vi "SCADA.vi"() -> ()   [LabVIEW 2014]
uses:
  <vilib>/platform/TimedLoop/XDataNode/XDataNode.xnode
  <vilib>/Platform/TimedLoop/XDataNode/nitl_modes.ctl
  <vilib>/Platform/TimedLoop/XDataNode/XDNodeRunTimeDep.lvlib
  <vilib>/Platform/TimedLoop/XDataNode/wakeup.ctl
  <vilib>/Platform/TimedLoop/XDataNode/timing_clust.ctl
panel:
  out "Hand_Error":bool
  out "Tasks":string
  out "State":string
  in  "HAND/AUTO":bool=TRUE
  in  "EMERGENCY ON/OFF":bool
  out "Fault":bool
  in  "ACK FAULT":bool
  in  "PUMPS OFF":bool
  in  "PUMPS ON":bool
  in  "SYSTEM OFF":bool
  in  "SYSTEM ON":bool
  out "error IO":errorcluster
  in  "error in (no error)":errorcluster
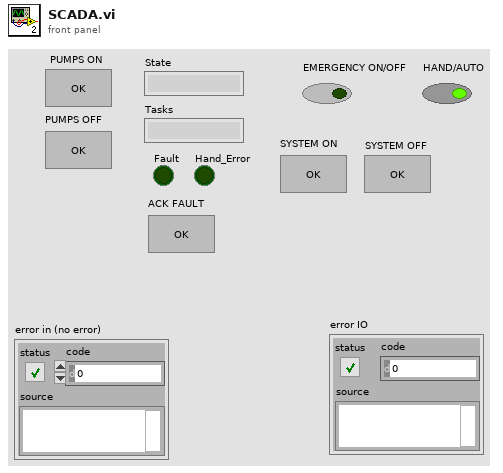
[diagram p1: front panel]
types:
  T1 = typedef "XDNodeRunTimeDep.lvlib/timing_clust.ctl" = cluster{"Expected End [f-1]":u64, "Actual End [f-1]":u64, "Finished Late? [f-1]":bool, "Expected End [i-1]":u64, "Actual End [i-1]":u64, "Finished Late? [i-1]":bool, "Expected Start [i]":u64, "Actual Start [i]":u64, "Expected Start [f]":u64, "Actual Start [f]":u64, "Source Name":string, "Structure Name":string, "Period":i64, "Deadline":i64, "Offset":i64, "Start":i64, "Priority":i32, "Timeout":i32, "Mode":T2, "Wakeup Reason":T3, "Error":errorcluster, "Source Type":string, "Secondary Source Type":string, "Global End Time":u64, "Global Start Time":u64, "Frame Duration":u64, "Iteration Duration":u64, "Assigned CPU":i32, "I/O Scan Engine Mode":u32}
  T2 = typedef "XDNodeRunTimeDep.lvlib/nitl_modes.ctl" = enum32{"No Change", "Process missed periods, maintain original phase", "Discard missed periods, maintain original phase", "Process missed periods, ignore original phase", "Discard missed periods, ignore original phase"}
  T3 = typedef "XDNodeRunTimeDep.lvlib/wakeup.ctl" = enum32{"Normal", "Aborted", "Asynchronous wakeup", "Timing source error", "Timed loop error", "Timeout"}
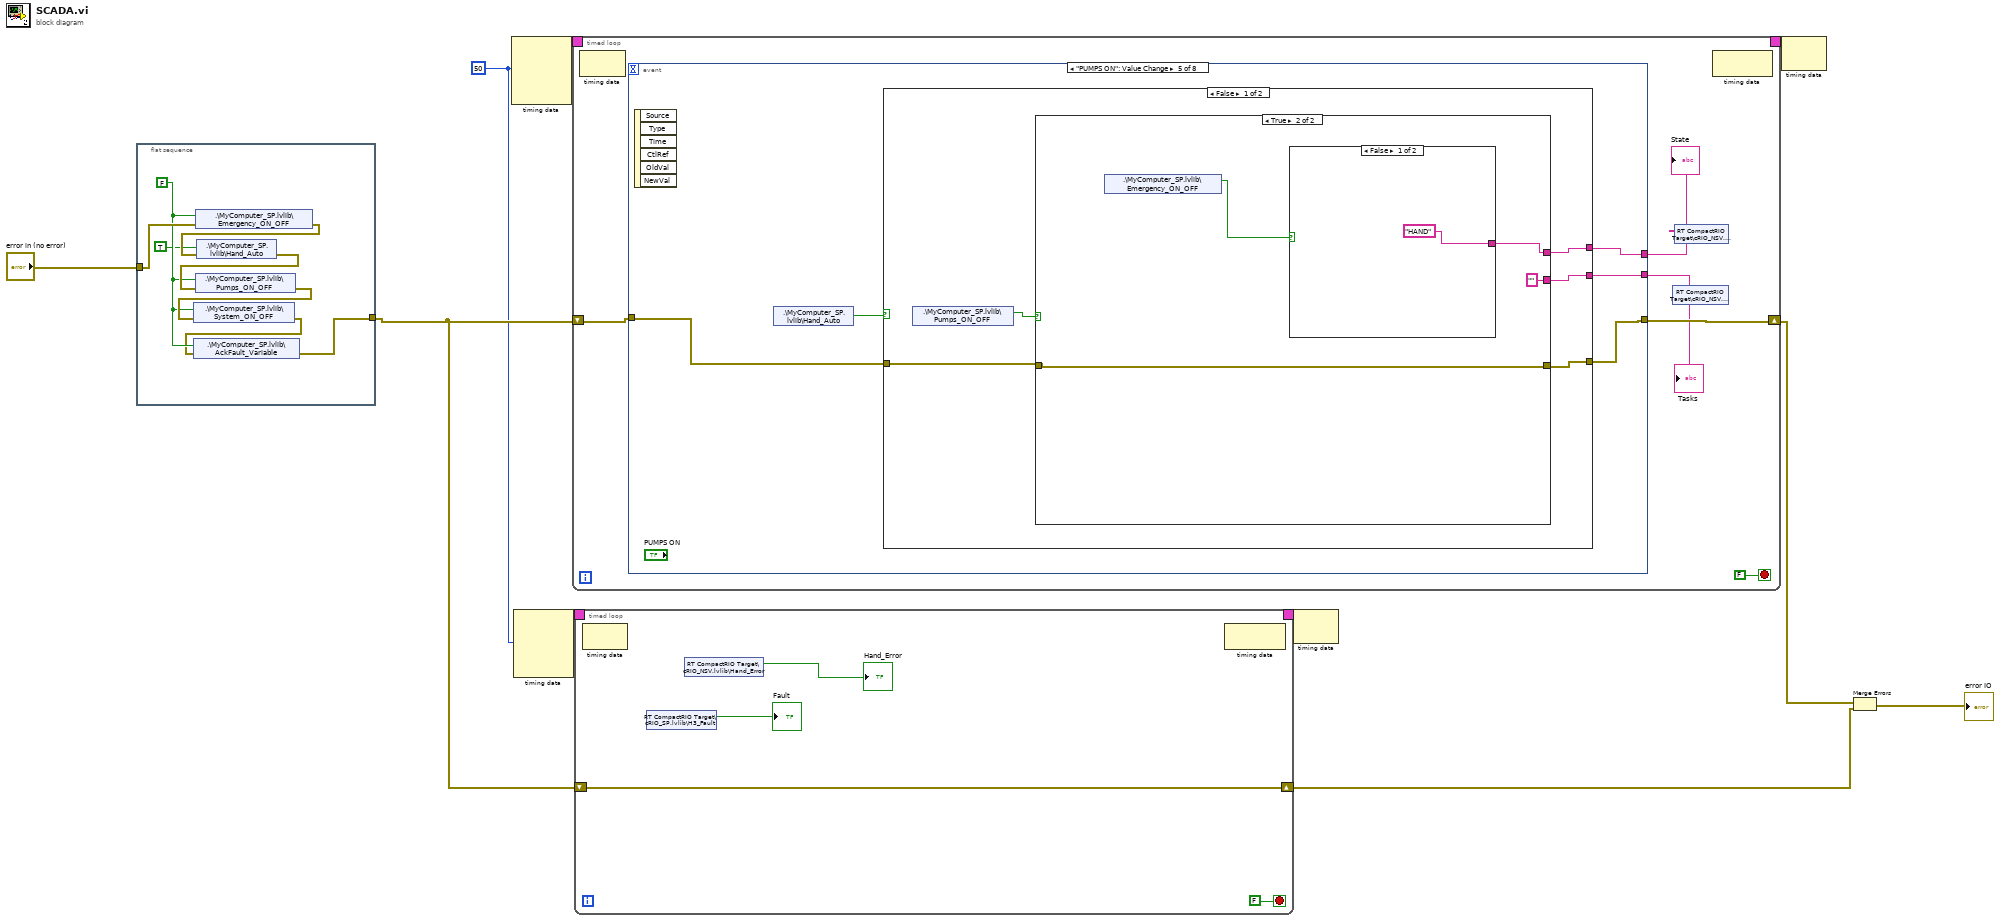
[diagram p0: block diagram]
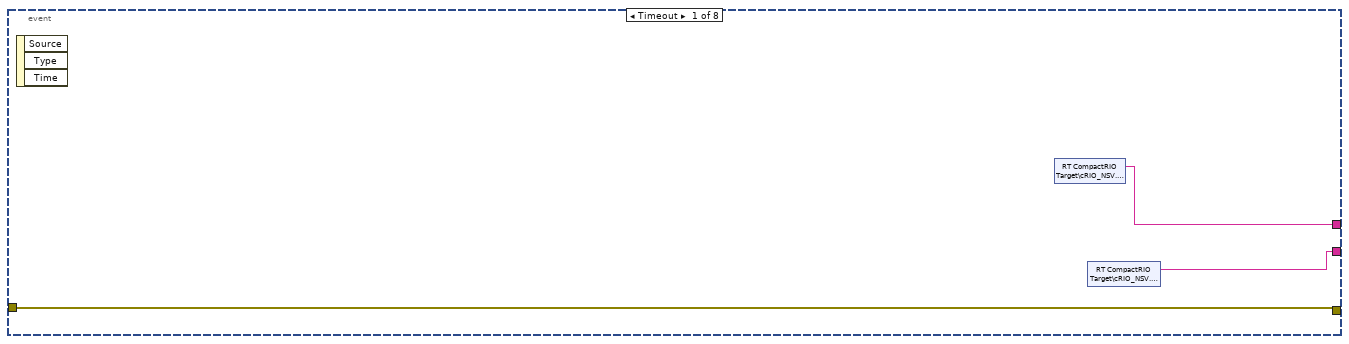
[diagram p2: hidden frame]
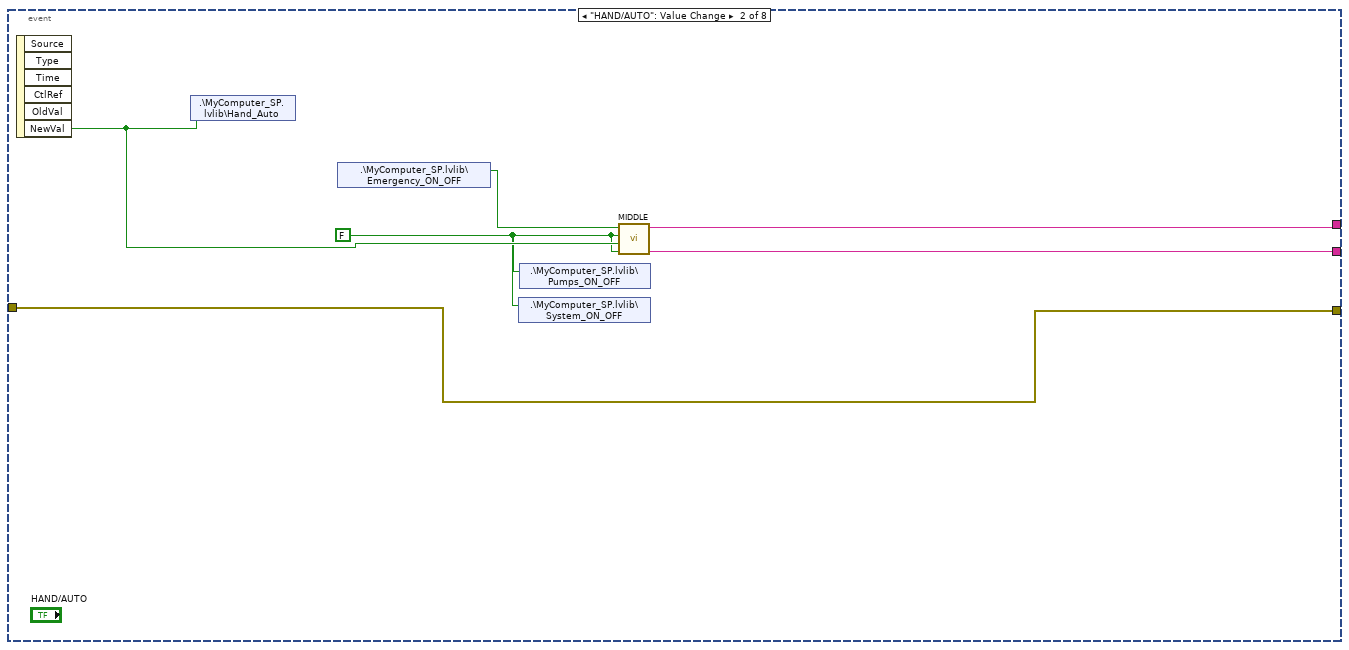
[diagram p3: hidden frame]
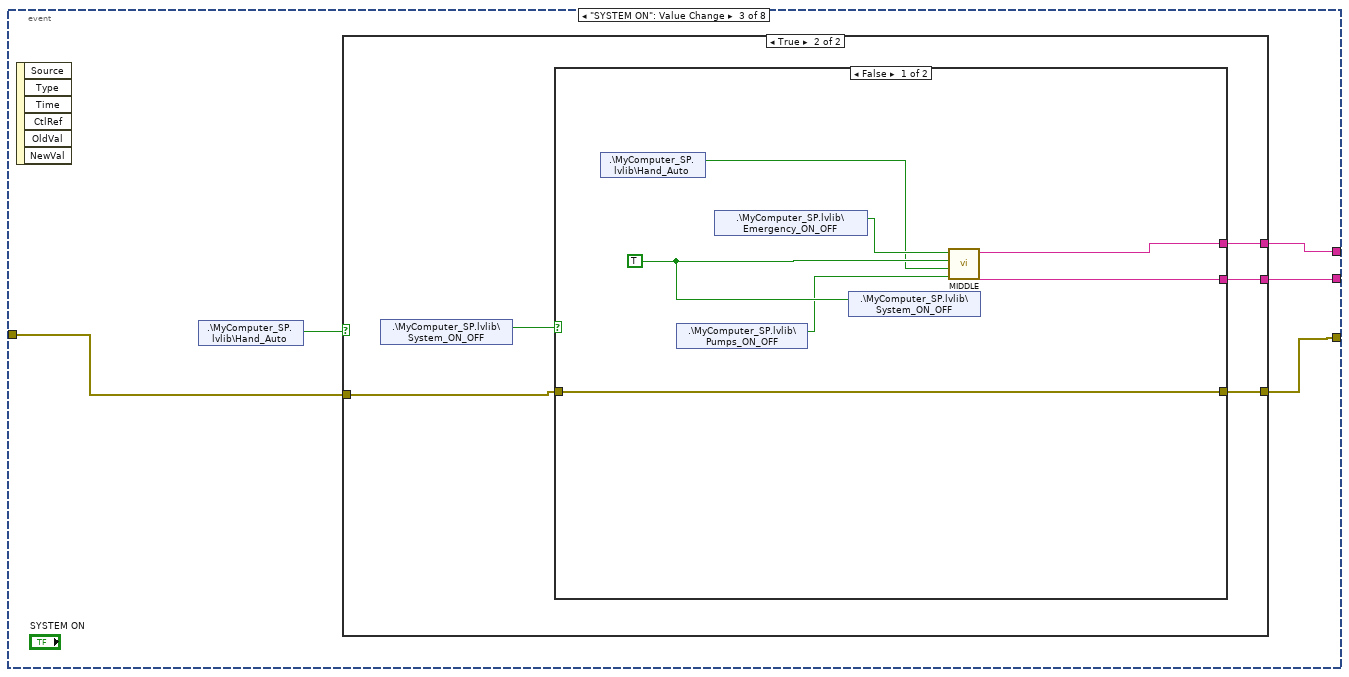
[diagram p4: hidden frame]
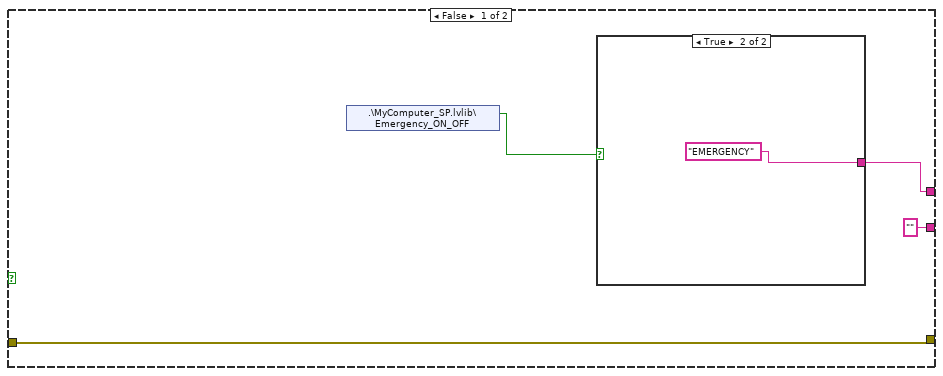
[diagram p5: hidden frame]
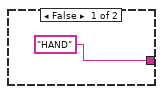
[diagram p6: hidden frame]
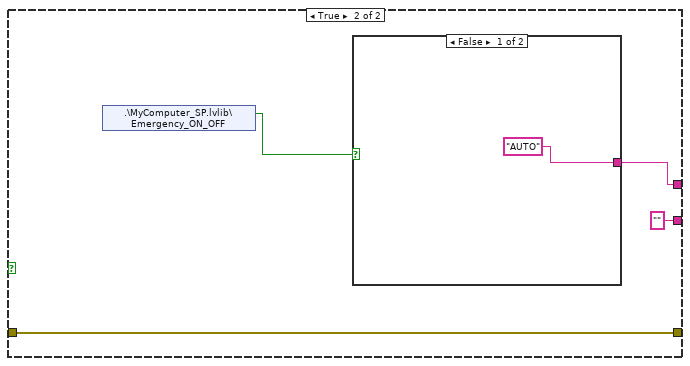
[diagram p7: hidden frame]
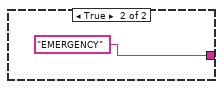
[diagram p8: hidden frame]
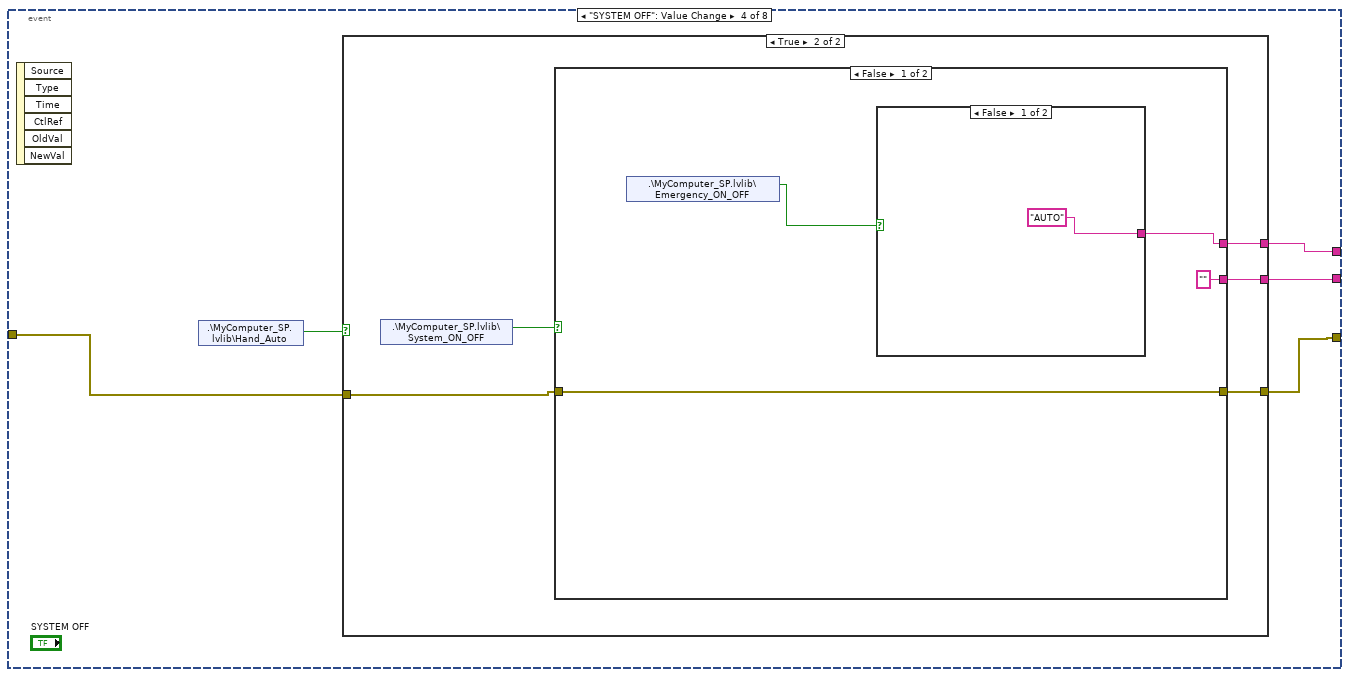
[diagram p9: hidden frame]
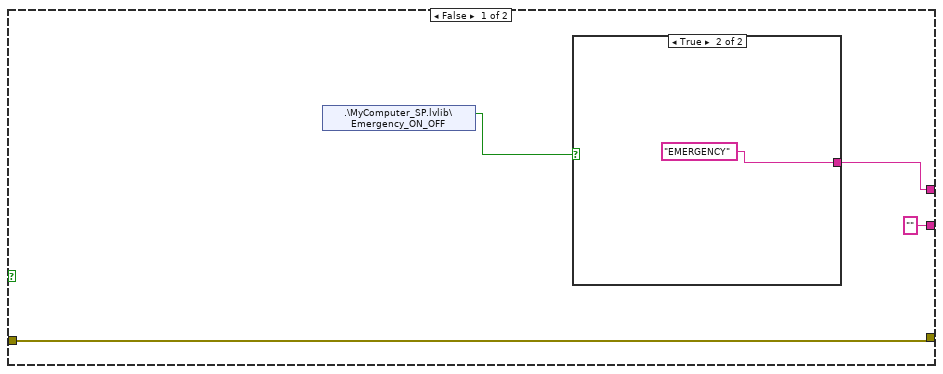
[diagram p10: hidden frame]
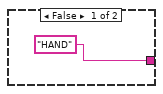
[diagram p11: hidden frame]
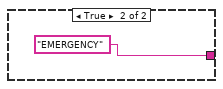
[diagram p12: hidden frame]
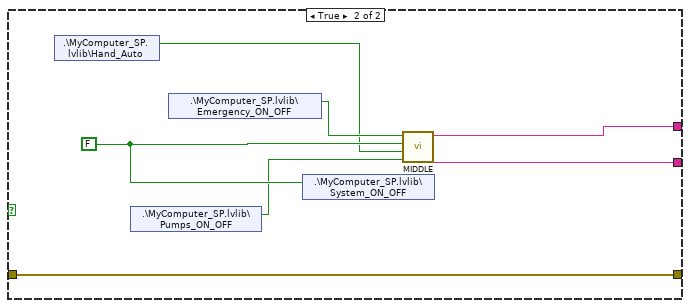
[diagram p13: hidden frame]
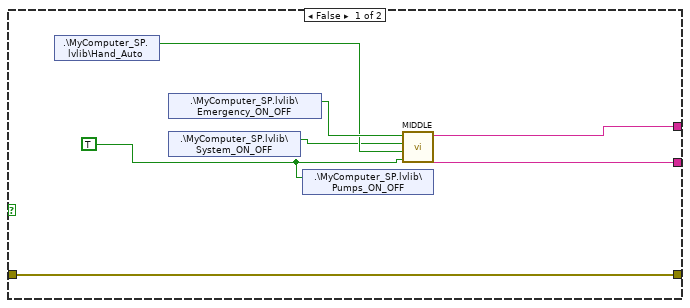
[diagram p14: hidden frame]
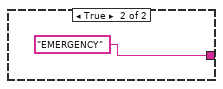
[diagram p15: hidden frame]
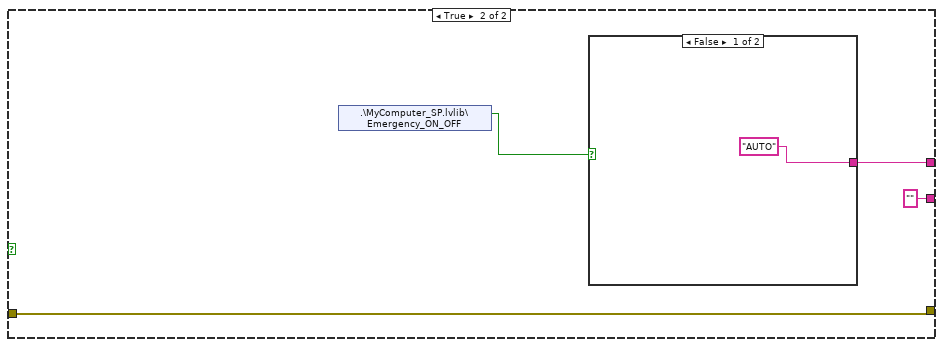
[diagram p16: hidden frame]
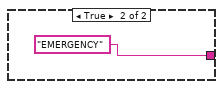
[diagram p17: hidden frame]
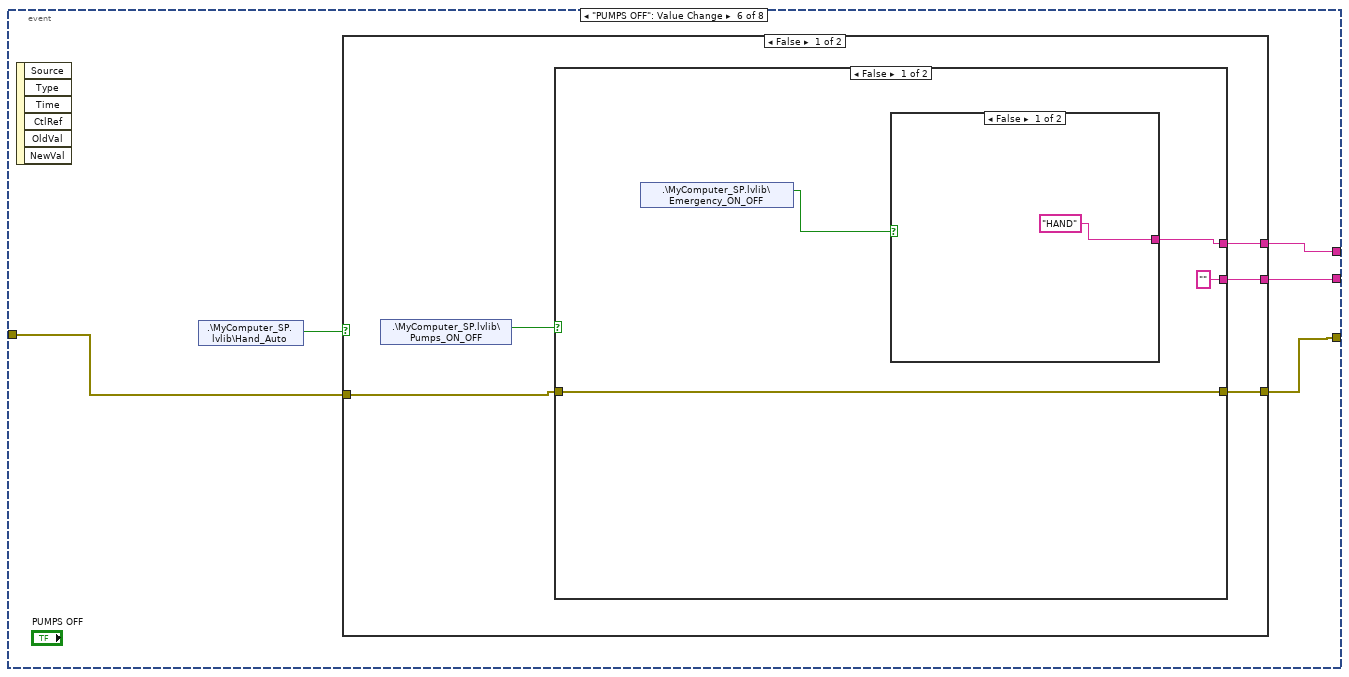
[diagram p18: hidden frame]
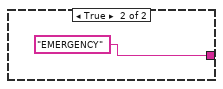
[diagram p19: hidden frame]
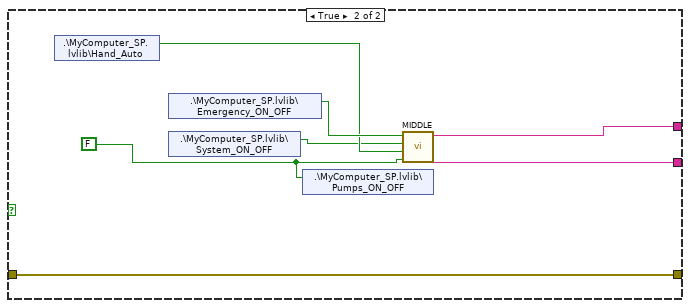
[diagram p20: hidden frame]
diagram:
  w1 = i64 50 ("Period")
  n1 = flat-sequence {
    tunnel: "error in (no error)" -> [w18]
    tunnel: [w12] -> w6
    frame #0 {
      w14 = FALSE
      n2 = shared-variable ".\\MyComputer_SP.lvlib\\Emergency_ON_OFF"(w14, error in=w18) -> (error out=w17:errorcluster)
      n3 = shared-variable ".\\MyComputer_SP.lvlib\\Hand_Auto"(TRUE, error in=w17) -> (error out=w16:errorcluster)
      n4 = shared-variable ".\\MyComputer_SP.lvlib\\Pumps_ON_OFF"(w14, error in=w16) -> (error out=w15:errorcluster)
      n5 = shared-variable ".\\MyComputer_SP.lvlib\\System_ON_OFF"(w14, error in=w15) -> (error out=w13:errorcluster)
      n6 = shared-variable ".\\MyComputer_SP.lvlib\\AckFault_Variable"(w14, error in=w13) -> (error out=w12:errorcluster)
    }
  }
  n7 = node-c288(w1) -> (w5:T1)  [unwired: 3 in]
  n8 = node-c288(w1) -> (w3:T1)  [unwired: 3 in]
  n9 = timed-loop {
    shift-right: [w21] -> w9
    shift-left: w6 -> [w22]
    timing: w5 -> [_]
    timing-out: [_] -> w4
    stop <- FALSE stop-if-true
    n10 = node-c288() -> ()  [unwired: 1 in, 1 out]
    n11 = event shown="[4] \"PUMPS ON\": Value Change" {
      selector: _ -> [_ _ _ _ _ _ _ _]
      dyn-events: _ -> [_ _ _ _ _ _ _ _]
      timeout: _ -> [_ _ _ _ _ _ _ _]
      tunnel: w22 -> [w26 w29 w36 w65 w94 w123 w152 w169]
      tunnel: [w28 w31 w37 w66 w95 w124 w154 w167] -> w20
      tunnel: [w27 w30 w38 w67 w96 w125 w153 w166] -> w19
      tunnel: [w26 w29 w35 w64 w93 w122 w151 w168] -> w21
      event Timeout {
        n12 = event-data() -> ()  [unwired: 1 in, 3 out]
        n13 = shared-variable "RT CompactRIO Target\\cRIO_NSV.lvlib\\State"() -> (w28:string)  [unwired: 1 in, 1 out]
        n14 = shared-variable "RT CompactRIO Target\\cRIO_NSV.lvlib\\Tasks"() -> (w27:string)  [unwired: 1 in, 1 out]
      }
      event "HAND/AUTO": Value Change {
        w32 = FALSE
        n15 = event-data() -> ("NewVal"=w33:bool)  [unwired: 1 in, 5 out]
        n16 = shared-variable ".\\MyComputer_SP.lvlib\\Hand_Auto"(w33) -> ()  [unwired: 1 in, 1 out]
        n17 = shared-variable ".\\MyComputer_SP.lvlib\\Emergency_ON_OFF"() -> (w34:bool)  [unwired: 1 in, 1 out]
        n18 = shared-variable ".\\MyComputer_SP.lvlib\\System_ON_OFF"(w32) -> ()  [unwired: 1 in, 1 out]
        n19 = shared-variable ".\\MyComputer_SP.lvlib\\Pumps_ON_OFF"(w32) -> ()  [unwired: 1 in, 1 out]
        n20 = call "MIDDLE.vi"("PUMPS ON/OFF"=w32, "HAND/AUTO"=w33, "SYSTEM ON/OFF"=w32, "EMERGENCY ON/OFF"=w34) -> ("Tasks"=w30:string, "State"=w31:string)  [unwired: 6 in]
      }
      event "SYSTEM ON": Value Change {
        n21 = event-data() -> ()  [unwired: 1 in, 6 out]
        n22 = shared-variable ".\\MyComputer_SP.lvlib\\Hand_Auto"() -> (w39:bool)  [unwired: 1 in, 1 out]
        n23 = case shown="True" w39 {
          tunnel: ["" ("String") w49] -> w38
          tunnel: [w40 w48] -> w37
          tunnel: w36 -> [w43 w47]
          tunnel: [w43 w46] -> w35
          frame False {
            n24 = shared-variable ".\\MyComputer_SP.lvlib\\Emergency_ON_OFF"() -> (w41:bool)  [unwired: 1 in, 1 out]
            n25 = case shown="True" w41 {
              tunnel: ["HAND" ("String") "EMERGENCY" ("String")] -> w40
              frame False {
              }
              frame True {
              }
            }
          }
          frame True {
            n26 = shared-variable ".\\MyComputer_SP.lvlib\\System_ON_OFF"() -> (w50:bool)  [unwired: 1 in, 1 out]
            n27 = case shown="False" w50 {
              tunnel: [w52 "" ("Tasks")] -> w49
              tunnel: [w53 w58] -> w48
              tunnel: w47 -> [w51 w61]
              tunnel: [w51 w61] -> w46
              frame False {
                w56 = TRUE ("SYSTEM ON/OFF")
                n28 = shared-variable ".\\MyComputer_SP.lvlib\\Hand_Auto"() -> (w54:bool)  [unwired: 1 in, 1 out]
                n29 = shared-variable ".\\MyComputer_SP.lvlib\\Pumps_ON_OFF"() -> (w55:bool)  [unwired: 1 in, 1 out]
                n30 = shared-variable ".\\MyComputer_SP.lvlib\\Emergency_ON_OFF"() -> (w57:bool)  [unwired: 1 in, 1 out]
                n31 = shared-variable ".\\MyComputer_SP.lvlib\\System_ON_OFF"(w56) -> ()  [unwired: 1 in, 1 out]
                n32 = call "MIDDLE.vi"("PUMPS ON/OFF"=w55, "HAND/AUTO"=w54, "SYSTEM ON/OFF"=w56, "EMERGENCY ON/OFF"=w57) -> ("Tasks"=w52:string, "State"=w53:string)  [unwired: 6 in]
              }
              frame True {
                n33 = shared-variable ".\\MyComputer_SP.lvlib\\Emergency_ON_OFF"() -> (w59:bool)  [unwired: 1 in, 1 out]
                n34 = case shown="False" w59 {
                  tunnel: ["AUTO" ("String") "EMERGENCY" ("String")] -> w58
                  frame False {
                  }
                  frame True {
                  }
                }
              }
            }
          }
        }
      }
      event "SYSTEM OFF": Value Change {
        n35 = event-data() -> ()  [unwired: 1 in, 6 out]
        n36 = shared-variable ".\\MyComputer_SP.lvlib\\Hand_Auto"() -> (w68:bool)  [unwired: 1 in, 1 out]
        n37 = case shown="True" w68 {
          tunnel: ["" ("Tasks") w78] -> w67
          tunnel: [w69 w77] -> w66
          tunnel: w65 -> [w72 w76]
          tunnel: [w72 w75] -> w64
          frame False {
            n38 = shared-variable ".\\MyComputer_SP.lvlib\\Emergency_ON_OFF"() -> (w70:bool)  [unwired: 1 in, 1 out]
            n39 = case shown="True" w70 {
              tunnel: ["HAND" ("String") "EMERGENCY" ("String")] -> w69
              frame False {
              }
              frame True {
              }
            }
          }
          frame True {
            n40 = shared-variable ".\\MyComputer_SP.lvlib\\System_ON_OFF"() -> (w79:bool)  [unwired: 1 in, 1 out]
            n41 = case shown="False" w79 {
              tunnel: ["" ("Tasks") w87] -> w78
              tunnel: [w80 w88] -> w77
              tunnel: w76 -> [w83 w86]
              tunnel: [w83 w86] -> w75
              frame False {
                n42 = shared-variable ".\\MyComputer_SP.lvlib\\Emergency_ON_OFF"() -> (w81:bool)  [unwired: 1 in, 1 out]
                n43 = case shown="False" w81 {
                  tunnel: ["AUTO" ("String") "EMERGENCY" ("String")] -> w80
                  frame False {
                  }
                  frame True {
                  }
                }
              }
              frame True {
                w91 = FALSE ("SYSTEM ON/OFF")
                n44 = shared-variable ".\\MyComputer_SP.lvlib\\Hand_Auto"() -> (w89:bool)  [unwired: 1 in, 1 out]
                n45 = shared-variable ".\\MyComputer_SP.lvlib\\Pumps_ON_OFF"() -> (w90:bool)  [unwired: 1 in, 1 out]
                n46 = shared-variable ".\\MyComputer_SP.lvlib\\Emergency_ON_OFF"() -> (w92:bool)  [unwired: 1 in, 1 out]
                n47 = shared-variable ".\\MyComputer_SP.lvlib\\System_ON_OFF"(w91) -> ()  [unwired: 1 in, 1 out]
                n48 = call "MIDDLE.vi"("PUMPS ON/OFF"=w90, "HAND/AUTO"=w89, "SYSTEM ON/OFF"=w91, "EMERGENCY ON/OFF"=w92) -> ("Tasks"=w87:string, "State"=w88:string)  [unwired: 6 in]
              }
            }
          }
        }
      }
      event "PUMPS ON": Value Change {
        n49 = event-data() -> ()  [unwired: 1 in, 6 out]
        n50 = shared-variable ".\\MyComputer_SP.lvlib\\Hand_Auto"() -> (w97:bool)  [unwired: 1 in, 1 out]
        n51 = case shown="False" w97 {
          tunnel: [w101 "" ("Tasks")] -> w96
          tunnel: [w100 w117] -> w95
          tunnel: w94 -> [w99 w119]
          tunnel: [w98 w119] -> w93
          frame False {
            n52 = shared-variable ".\\MyComputer_SP.lvlib\\Pumps_ON_OFF"() -> (w102:bool)  [unwired: 1 in, 1 out]
            n53 = case shown="True" w102 {
              tunnel: [w106 "" ("Tasks")] -> w101
              tunnel: [w107 w110] -> w100
              tunnel: w99 -> [w105 w113]
              tunnel: [w105 w113] -> w98
              frame False {
                w103 = TRUE ("SYSTEM ON/OFF")
                n54 = shared-variable ".\\MyComputer_SP.lvlib\\Hand_Auto"() -> (w108:bool)  [unwired: 1 in, 1 out]
                n55 = shared-variable ".\\MyComputer_SP.lvlib\\Emergency_ON_OFF"() -> (w109:bool)  [unwired: 1 in, 1 out]
                n56 = shared-variable ".\\MyComputer_SP.lvlib\\System_ON_OFF"() -> (w104:bool)  [unwired: 1 in, 1 out]
                n57 = shared-variable ".\\MyComputer_SP.lvlib\\Pumps_ON_OFF"(w103) -> ()  [unwired: 1 in, 1 out]
                n58 = call "MIDDLE.vi"("PUMPS ON/OFF"=w103, "HAND/AUTO"=w108, "SYSTEM ON/OFF"=w104, "EMERGENCY ON/OFF"=w109) -> ("Tasks"=w106:string, "State"=w107:string)  [unwired: 6 in]
              }
              frame True {
                n59 = shared-variable ".\\MyComputer_SP.lvlib\\Emergency_ON_OFF"() -> (w111:bool)  [unwired: 1 in, 1 out]
                n60 = case shown="False" w111 {
                  tunnel: ["HAND" ("String") "EMERGENCY" ("String")] -> w110
                  frame False {
                  }
                  frame True {
                  }
                }
              }
            }
          }
          frame True {
            n61 = shared-variable ".\\MyComputer_SP.lvlib\\Emergency_ON_OFF"() -> (w116:bool)  [unwired: 1 in, 1 out]
            n62 = case shown="False" w116 {
              tunnel: ["AUTO" ("String") "EMERGENCY" ("String")] -> w117
              frame False {
              }
              frame True {
              }
            }
          }
        }
      }
      event "PUMPS OFF": Value Change {
        n63 = event-data() -> ()  [unwired: 1 in, 6 out]
        n64 = shared-variable ".\\MyComputer_SP.lvlib\\Hand_Auto"() -> (w126:bool)  [unwired: 1 in, 1 out]
        n65 = case shown="False" w126 {
          tunnel: [w130 "" ("Tasks")] -> w125
          tunnel: [w129 w146] -> w124
          tunnel: w123 -> [w128 w148]
          tunnel: [w127 w148] -> w122
          frame False {
            n66 = shared-variable ".\\MyComputer_SP.lvlib\\Pumps_ON_OFF"() -> (w131:bool)  [unwired: 1 in, 1 out]
            n67 = case shown="False" w131 {
              tunnel: ["" ("Tasks") w141] -> w130
              tunnel: [w132 w142] -> w129
              tunnel: w128 -> [w135 w140]
              tunnel: [w135 w140] -> w127
              frame False {
                n68 = shared-variable ".\\MyComputer_SP.lvlib\\Emergency_ON_OFF"() -> (w133:bool)  [unwired: 1 in, 1 out]
                n69 = case shown="False" w133 {
                  tunnel: ["HAND" ("String") "EMERGENCY" ("String")] -> w132
                  frame False {
                  }
                  frame True {
                  }
                }
              }
              frame True {
                w138 = FALSE ("SYSTEM ON/OFF")
                n70 = shared-variable ".\\MyComputer_SP.lvlib\\Hand_Auto"() -> (w143:bool)  [unwired: 1 in, 1 out]
                n71 = shared-variable ".\\MyComputer_SP.lvlib\\Emergency_ON_OFF"() -> (w144:bool)  [unwired: 1 in, 1 out]
                n72 = shared-variable ".\\MyComputer_SP.lvlib\\System_ON_OFF"() -> (w139:bool)  [unwired: 1 in, 1 out]
                n73 = shared-variable ".\\MyComputer_SP.lvlib\\Pumps_ON_OFF"(w138) -> ()  [unwired: 1 in, 1 out]
                n74 = call "MIDDLE.vi"("PUMPS ON/OFF"=w138, "HAND/AUTO"=w143, "SYSTEM ON/OFF"=w139, "EMERGENCY ON/OFF"=w144) -> ("Tasks"=w141:string, "State"=w142:string)  [unwired: 6 in]
              }
            }
          }
          frame True {
            n75 = shared-variable ".\\MyComputer_SP.lvlib\\Emergency_ON_OFF"() -> (w145:bool)  [unwired: 1 in, 1 out]
            n76 = case shown="True" w145 {
              tunnel: ["AUTO" ("String") "EMERGENCY" ("String")] -> w146
              frame False {
              }
              frame True {
              }
            }
          }
        }
      }
      event "EMERGENCY ON/OFF": Value Change {
        n77 = event-data() -> ("NewVal"=w155:bool)  [unwired: 1 in, 5 out]
        n78 = shared-variable ".\\MyComputer_SP.lvlib\\Emergency_ON_OFF"(w155) -> ()  [unwired: 1 in, 1 out]
        n79 = case shown="False" w155 {
          selector: w155 -> [_ w165]
          tunnel: [w157 w162] -> w154
          tunnel: [w158 w161] -> w153
          tunnel: w152 -> [w156 w160]
          tunnel: [w156 w160] -> w151
          frame False {
            n80 = shared-variable "RT CompactRIO Target\\cRIO_NSV.lvlib\\State"() -> (w157:string)  [unwired: 1 in, 1 out]
            n81 = shared-variable "RT CompactRIO Target\\cRIO_NSV.lvlib\\Tasks"() -> (w158:string)  [unwired: 1 in, 1 out]
          }
          frame True {
            w159 = TRUE ("AckFault_Variable")
            w164 = FALSE
            n82 = shared-variable ".\\MyComputer_SP.lvlib\\Hand_Auto"() -> (w163:bool)  [unwired: 1 in, 1 out]
            n83 = shared-variable ".\\MyComputer_SP.lvlib\\System_ON_OFF"(w164) -> ()  [unwired: 1 in, 1 out]
            n84 = call "MIDDLE.vi"("PUMPS ON/OFF"=w164, "HAND/AUTO"=w163, "SYSTEM ON/OFF"=w164, "EMERGENCY ON/OFF"=w165) -> ("Tasks"=w161:string, "State"=w162:string)  [unwired: 6 in]
            n85 = shared-variable ".\\MyComputer_SP.lvlib\\Pumps_ON_OFF"(w164) -> ()  [unwired: 1 in, 1 out]
            n86 = shared-variable ".\\MyComputer_SP.lvlib\\AckFault_Variable"(w159) -> ()  [unwired: 1 in, 1 out]
            n87 = shared-variable "RT CompactRIO Target\\cRIO_SP.lvlib\\H3_Fault"(w159) -> ()  [unwired: 1 in, 1 out]
          }
        }
      }
      event "ACK FAULT": Value Change {
        n88 = event-data() -> ()  [unwired: 1 in, 6 out]
        n89 = shared-variable ".\\MyComputer_SP.lvlib\\Emergency_ON_OFF"() -> (w170:bool)  [unwired: 1 in, 1 out]
        n90 = case shown="False" w170 {
          tunnel: w169 -> [w173 w177]
          tunnel: [w173 w176] -> w168
          tunnel: [w172 w175] -> w167
          tunnel: [w171 w174] -> w166
          frame True {
            n91 = shared-variable "RT CompactRIO Target\\cRIO_NSV.lvlib\\State"() -> (w172:string)  [unwired: 1 in, 1 out]
            n92 = shared-variable "RT CompactRIO Target\\cRIO_NSV.lvlib\\Tasks"() -> (w171:string)  [unwired: 1 in, 1 out]
          }
          frame False {
            n93 = shared-variable ".\\MyComputer_SP.lvlib\\AckFault_Variable"() -> (w178:bool)  [unwired: 1 in, 1 out]
            n94 = case shown="True" w178 {
              tunnel: w177 -> [w181 w187]
              tunnel: [w181 w187] -> w176
              tunnel: [w180 w186] -> w175
              tunnel: [w179 w185] -> w174
              frame False {
                n95 = shared-variable "RT CompactRIO Target\\cRIO_NSV.lvlib\\Tasks"() -> (w179:string)  [unwired: 1 in, 1 out]
                n96 = shared-variable "RT CompactRIO Target\\cRIO_NSV.lvlib\\State"() -> (w180:string)  [unwired: 1 in, 1 out]
              }
              frame True {
                w183 = FALSE
                w182 = FALSE ("AckFault_Variable")
                n97 = shared-variable ".\\MyComputer_SP.lvlib\\Hand_Auto"() -> (w184:bool)  [unwired: 1 in, 1 out]
                n98 = call "MIDDLE.vi"("PUMPS ON/OFF"=w183, "HAND/AUTO"=w184, "SYSTEM ON/OFF"=w183, "EMERGENCY ON/OFF"=w183) -> ("Tasks"=w185:string, "State"=w186:string)  [unwired: 6 in]
                n99 = shared-variable ".\\MyComputer_SP.lvlib\\AckFault_Variable"(w182) -> ()  [unwired: 1 in, 1 out]
                n100 = shared-variable "RT CompactRIO Target\\cRIO_SP.lvlib\\H3_Fault"(w182) -> ()  [unwired: 1 in, 1 out]
              }
            }
          }
        }
      }
    }
    "State" <- w20
    "Tasks" <- w19
    n101 = shared-variable "RT CompactRIO Target\\cRIO_NSV.lvlib\\Tasks"(w19) -> ()  [unwired: 1 in, 1 out]
    n102 = shared-variable "RT CompactRIO Target\\cRIO_NSV.lvlib\\State"(w20) -> ()  [unwired: 1 in, 1 out]
    n103 = node-c288() -> ()  [unwired: 1 in, 1 out]
  }
  n104 = timed-loop {
    shift-right: [w191] -> w7
    shift-left: w6 -> [w191]
    timing: w3 -> [_]
    timing-out: [_] -> w2
    stop <- FALSE stop-if-true
    n105 = node-c288() -> ()  [unwired: 1 in, 1 out]
    n106 = shared-variable "RT CompactRIO Target\\cRIO_SP.lvlib\\H3_Fault"() -> (→"Fault":bool)  [unwired: 1 in, 1 out]
    n107 = shared-variable "RT CompactRIO Target\\cRIO_NSV.lvlib\\Hand_Error"() -> (→"Hand_Error":bool)  [unwired: 1 in, 1 out]
    n108 = node-c288() -> ()  [unwired: 1 in, 1 out]
  }
  n109 = node-c288(w2) -> ()  [unwired: 1 out]
  n110 = node-c288(w4) -> ()  [unwired: 1 out]
  n111 = Merge Errors(w9, w7) -> (→"error IO":errorcluster)
